vi "Configure Safety Settings.vi"(6 "Safety Limits":T2={"Temperature Limit (C)"=80, "Low Voltage Limit (V)"=5.0, "High Voltage Limit (V)"=25.0, "Maximum Torque%"=100.0}, 8 "error in (no error)":errorcluster, 9 "Alarm Settings":cluster{"LED Alarm":T1, "Shutdown Alarm":T1}={"LED Alarm"={"Input Voltage"=TRUE, "Angle Limit"=FALSE, "Overheating "=TRUE, "Range"=FALSE, "Checksum"=FALSE, "Overload"=FALSE, "Instruction"=FALSE}, "Shutdown Alarm"={"Input Voltage"=TRUE, "Angle Limit"=FALSE, "Overheating "=TRUE, "Range"=FALSE, "Checksum"=FALSE, "Overload"=FALSE, "Instruction"=FALSE}}, 10 "Motor ID (0)":u8, 11 "Dynamixel Motor in":refnum<class "Dynamixel Motor.lvclass">) -> (0 "error out":errorcluster, 3 "Dynamixel Motor out":refnum<class "Dynamixel Motor.lvclass">)   [LabVIEW 2016, in "Dynamixel Motor.lvclass"]
doc: "Sets limits for the temperature, voltage, and torque for the motor as well as the action to take for status errors for: temperature, overload, angle limit, checksum, etc."
uses:
  <instrlib>/Dynamixel Motor/HAIOL/Dynamixel Motor.lvclass
  <instrlib>/Dynamixel Motor/Public/Motor Operation/Low Level/Alarm Setting.ctl
  <instrlib>/Dynamixel Motor/Dynamixel Motor.lvlib
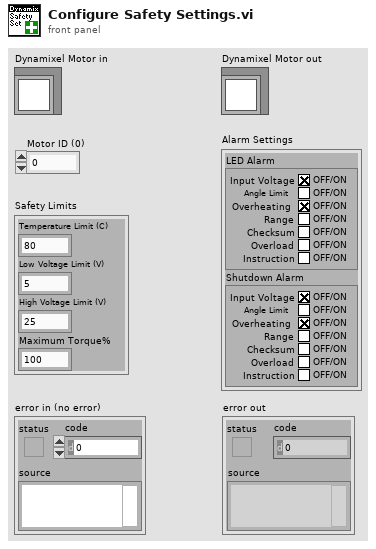
[diagram p1: front panel]
types:
  T1 = typedef "Dynamixel Motor.lvlib/Alarm Setting.ctl" = cluster{"Input Voltage":bool, "Angle Limit":bool, "Overheating ":bool, "Range":bool, "Checksum":bool, "Overload":bool, "Instruction":bool}
  T2 = cluster{"Temperature Limit (C)":u8, "Low Voltage Limit (V)":dbl, "High Voltage Limit (V)":dbl, "Maximum Torque%":dbl}
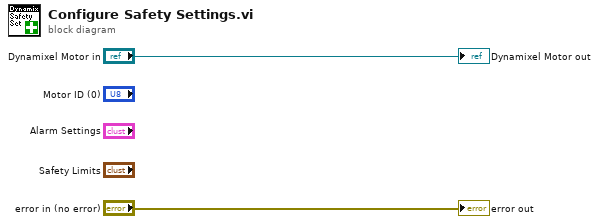
[diagram p0: block diagram]
diagram:
  "error out" <- "error in (no error)"
  "Dynamixel Motor out" <- "Dynamixel Motor in"
